vi "CheckAndCreateDirectory.vi"(0 "Path IN":path) -> (4 "Path OUT":path, 8 "Exists?":bool, 15 "Created?":bool)   [LabVIEW 2011]
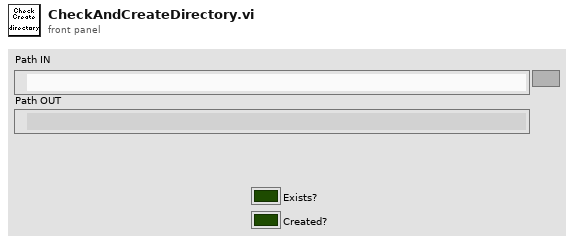
[diagram p1: front panel]
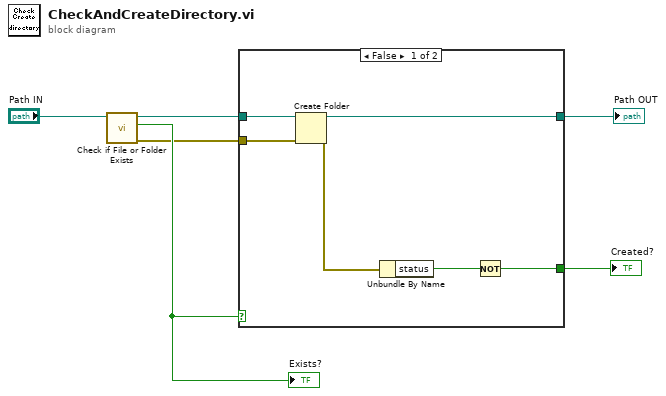
[diagram p0: block diagram]
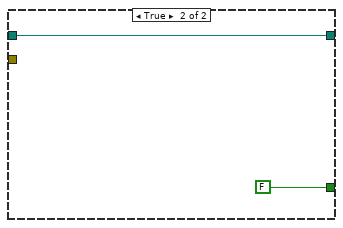
[diagram p2: hidden frame]
diagram:
  n1 = call <vilib>:"Check if File or Folder Exists.vi"("path"="Path IN") -> ("error out"=w2:errorcluster, "file or folder exists?"=w5:bool, "dup path"=w4:path)  [unwired: 8 in]
  "Exists?" <- w5
  n2 = case shown="False" w5 {
    tunnel: [w7 w14] -> w3
    tunnel: w4 -> [w12 w14]
    tunnel: w2 -> [w11 _]
    tunnel: [w8 FALSE] -> w1
    frame False {
      n3 = Create Folder(path (use dialog)=w12, error in=w11) -> (created path=w7:path, error out=w10:errorcluster)  [unwired: 1 in, 1 out]
      n4 = Unbundle By Name(w10) -> ("status"=w9:bool)
      n5 = Not(x=w9) -> (.not. x?=w8:bool)
    }
    frame True {
    }
  }
  "Created?" <- w1
  "Path OUT" <- w3
